vi "UTL_Read Controller Status.vi"(8 "error out":errorcluster) -> (0 "error out 2":errorcluster, 2 "Recipe":u16, 3 "Running Status":string)   [LabVIEW 2022 SP3]
uses:
  <vilib>/Plasmionique/MB Master/MB Master.lvlib
  Variable global de carga.vi
  <vilib>/Plasmionique/MB Master/MB_Master_Serial/MB_Master_Serial.lvclass
  C:/Program Files (x86)/National Instruments/LabVIEW 2022/vi.lib/Plasmionique/MB Master/MB_Master/MB_Master.lvclass
  C:/Program Files (x86)/National Instruments/LabVIEW 2022/vi.lib/Plasmionique/MB Master/MB_Master_Serial/MB_Master_Serial.lvclass
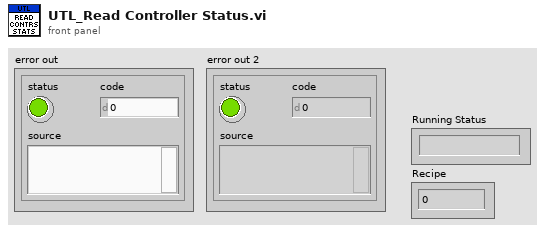
[diagram p1: front panel]
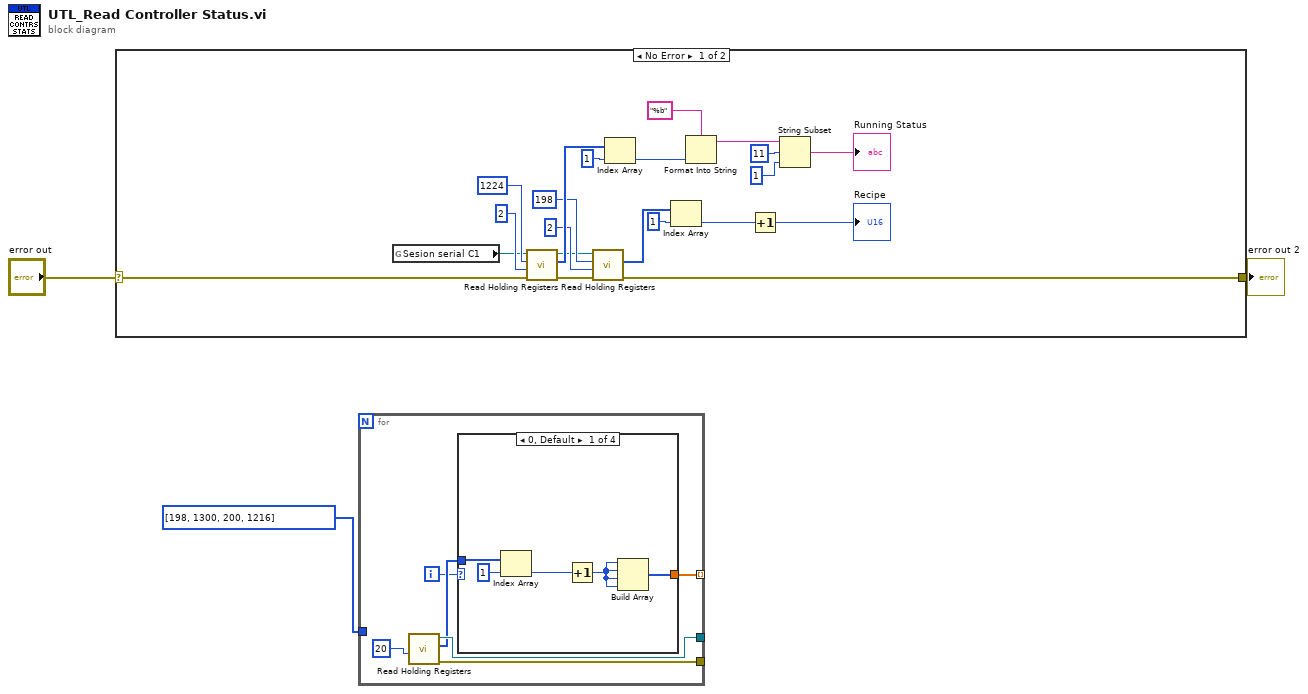
[diagram p0: block diagram]
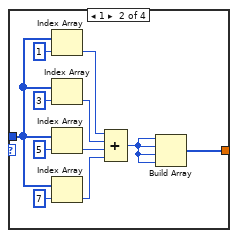
[diagram p2: hidden frame]
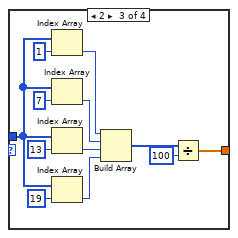
[diagram p3: hidden frame]
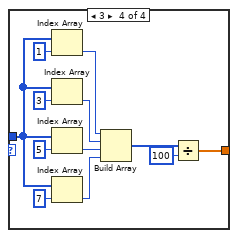
[diagram p4: hidden frame]
diagram:
  n1 = case shown="No Error" "error out" {
    selector: "error out" -> [w6 w25]
    tunnel: [w5 w25] -> w2
    frame No Error {
      n2 = global read "Variable global de carga.vi" "Sesion serial C1"() -> (w4:refnum<class "MB_Master_Serial.lvclass">)
      n3 = call <vilib>:"Read Holding Registers.vi"("error in (no error)"=w6, "quantity"=u16 2, "starting address"=1224, "MB session in"=w4) -> ("error out"=w18:errorcluster, "Registers"=w20:u16[], "MB session in"=w13:refnum<class "MB_Master_Serial.lvclass">)  [unwired: 5 in]
      n4 = call <vilib>:"Read Holding Registers.vi"("error in (no error)"=w18, "quantity"=u16 2, "starting address"=u16 198, "MB session in"=w13) -> ("error out"=w5:errorcluster, "Registers"=w14:u16[])  [unwired: 5 in, 1 out]
      n5 = Index Array(array=w20, index=1) -> (element=w10:u16)
      n6 = Index Array(array=w14, index=1) -> (element=w12:u16)
      n7 = Format Into String(format string="%b", w10) -> (resulting string=w9:string)  [unwired: 2 in, 1 out]
      n8 = Increment(x=w12) -> (x+1=→"Recipe":u16)
      n9 = String Subset(string=w9, offset (0)=11, length (rest)=1 ("length (rest)")) -> (substring=→"Running Status":string)
    }
    frame Error {
    }
  }
  "error out 2" <- w2
  n10 = for {
    tunnel: i32[] [198, 1300, 200, 1216] -> [_]
    tunnel: [w29] -> _
    tunnel: [w30] -> _
    tunnel: [w26] -> _ mode=indexing
    i -> [w27]
    n11 = call <vilib>:"Read Holding Registers.vi"("quantity"=u16 20) -> ("error out"=w30:errorcluster, "Registers"=w28:u16[], "MB session out"=w29:refnum<class "MB_Master.lvclass">)  [unwired: 8 in]
    n12 = case shown="0, Default" w27 {
      tunnel: w28 -> [w36 w43 w55 w67]
      tunnel: [w32 w37 w48 w60] -> w26
      frame 0, Default {
        n13 = Index Array(array=w36, index=1) -> (element=w34:u16)
        n14 = Increment(x=w34) -> (x+1=w33:u16)
        n15 = Build Array(w33, w33, w33, w33) -> (w32:u16[])
      }
      frame 1 {
        n16 = Index Array(array=w43, index=1) -> (element=w42:u16)
        n17 = Index Array(array=w43, index=3) -> (element=w41:u16)
        n18 = Index Array(array=w43, index=5) -> (element=w40:u16)
        n19 = Index Array(array=w43, index=7) -> (element=w39:u16)
        n20 = Compound Arithmetic op=ADD(w42, w41, w40, w39) -> (w38:u16)
        n21 = Build Array(w38, w38, w38, w38) -> (w37:u16[])
      }
      frame 2 {
        n22 = Index Array(array=w55, index=1) -> (element=w54:u16)
        n23 = Index Array(array=w55, index=7) -> (element=w53:u16)
        n24 = Index Array(array=w55, index=13) -> (element=w52:u16)
        n25 = Index Array(array=w55, index=19) -> (element=w51:u16)
        n26 = Build Array(w54, w53, w52, w51) -> (w49:u16[])
        n27 = Divide(x=w49, y=100) -> (x/y=w48:dbl[])
      }
      frame 3 {
        n28 = Index Array(array=w67, index=1) -> (element=w66:u16)
        n29 = Index Array(array=w67, index=3) -> (element=w65:u16)
        n30 = Index Array(array=w67, index=5) -> (element=w64:u16)
        n31 = Index Array(array=w67, index=7) -> (element=w63:u16)
        n32 = Build Array(w66, w65, w64, w63) -> (w62:u16[])
        n33 = Divide(x=w62, y=100) -> (x/y=w60:dbl[])
      }
    }
  }
